vi "Engine Knocking Detection.vi"() -> ()   [LabVIEW 2023]
doc: "This example shows the application of arbitrary path decomposition in detecting engine knocking.\n\nAnalyzing the acoustic signals, or vibrations, of engines plays an important role in engine designing and testing. You can use the wavelet transform-based method to detect the knocking of an engine. In the example data, the knocking sound is merged in the noise. After processing the signal with wavelet-based arbitrary path decomposition and reconstruction, you can detect the knocking sound easily.\n\nThis example uses the WA Arbitrary Path Decomposition VI and the WA Arbitrary Path Reconstruction VI.\n\n<b>Instructions:</b>\n1) Run this VI.\n2) Observe how the engine knocking becomes obvious in the enhanced sound."
uses:
  <vilib>/addons/Wavelet Analysis/typedefs.llb/WA Data.ctl
  <vilib>/addons/Wavelet Analysis/discrete wavelet transform.llb/WA Arbitrary Path Decomposition (Waveform).vi
  <vilib>/addons/Wavelet Analysis/discrete wavelet transform.llb/WA Arbitrary Path Reconstruction (Waveform).vi
  <vilib>/addons/_Advanced Signal Processing/NI_AdvSigProcWA.lvlib
panel:
  out "aspt-left-top":bool
  in  "stop":bool
  in  "Path":string="11"
  in  "Wavelet":u16(ring) items=["db02"=0, "db03"=1, "db04"=2, "db05"=3, "db06"=4, "db07"=5, "db08"=6, "db09"=7, "db10"=8, "db11"=9, "db12"=10, "db13"=11, "db14"=12, "Haar"=13, "bior1_3"=14, "bior1_5"=15, "bior2_2"=16, "bior2_4"=17, "bior2_6"=18, "bior2_8"=19, "bior3_1"=20, "bior3_3"=21, "bior3_5"=22, "bior3_7"=23, "bior3_9"=24, "bior4_4 (FBI)"=25, "bior5_5"=38, "bior6_8"=39, "coif1"=26, "coif2"=27, "coif3"=28, "coif4"=29, "coif5"=30, "sym2"=31, "sym3"=32, "sym4"=33, "sym5"=34, "sym6"=35, "sym7"=36, "sym8"=37]
  out "Engine Knocking Sound":waveform(dbl)(graph)
  out "Enhanced Sound":waveform(dbl)(graph)
  # "Overview: Shows the application of arbitrary path decomposition in detecting engine knocking.\nRequirements: LabVIEW Full Development System, Advanced Signal Processing Toolkit\nInstructions: \n1. Run this VI.\n2. Observe how the engine knocking becomes obvious in the enhanced sound.\n3. Click Stop to stop the VI."
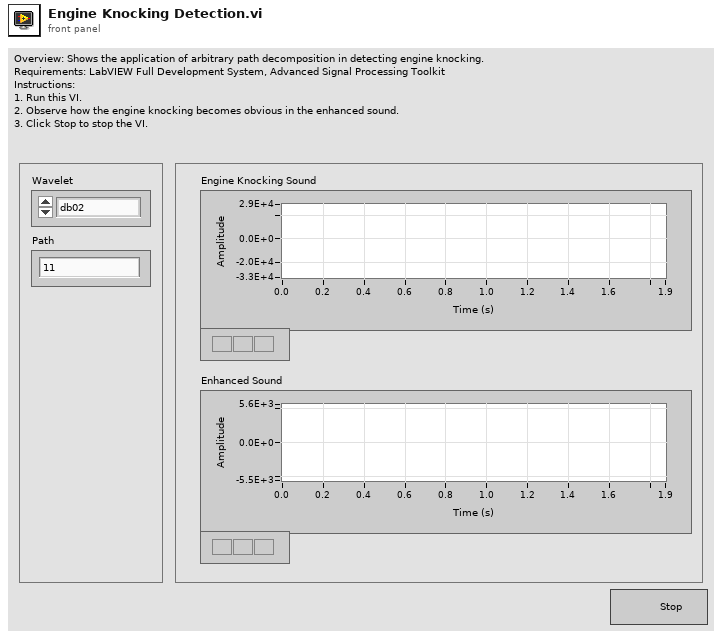
[diagram p1: front panel]
types:
  T1 = typedef "NI_AdvSigProcWA.lvlib/WA Data.ctl" = u16
  T2 = cluster{"coef":dbl[], "length":i32[], "residual path":string[]}
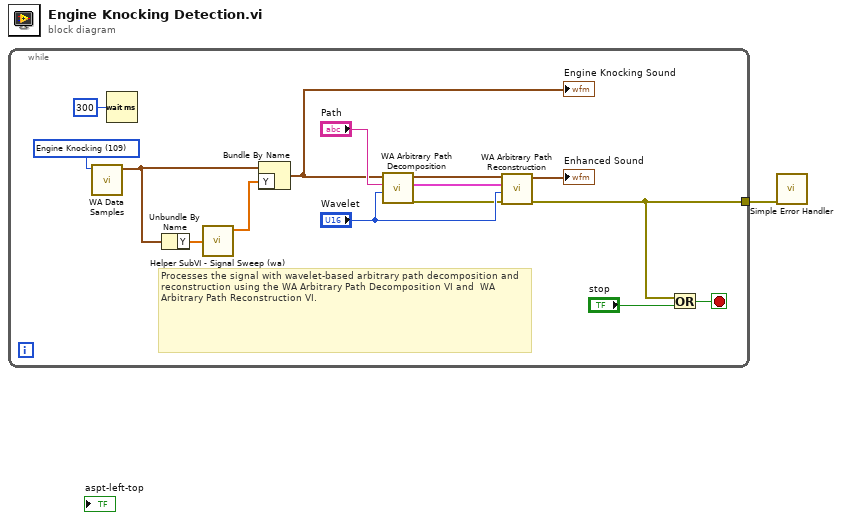
[diagram p0: block diagram]
diagram:
  n1 = while {
    tunnel: [w6] -> w1
    stop <- w9 stop-if-true
    w7 = T1 109 items=["1D Example Data"=100, "-"=101, "Doppler"=102, "HOP"=103, "TF Sine"=104, "Noisy Doppler"=105, "Sea Temperature"=106, "Sp500"=107, "Power Line"=108, "Engine Knocking"=109, "HeaviSine"=110, "Bumps"=111, "Blocks"=112, "Piece Regular"=113, "HypChirps"=114, "LinChirps"=115, "Chirps"=116, "Piece Polynomial"=117, "ECG"=131, "-"=118, "2D Example Data"=119, "-"=120, "Finger Print (Image)"=121, "Iris Flower (Image)"=122, "Mammogram (Image)"=123, "Lake (Image)"=127, "Two Can 1 (Image)"=132, "Two Can 2 (Image)"=133, "Camera Man (Image)"=134] ("data")
    # "Processes the signal with wavelet-based arbitrary path decomposition and reconstruction using the WA Arbitrary Path Decomposition VI and  WA Arbitrary Path Reconstruction VI."
    n2 = call <vilib>:"WA Data Samples.vi"("data"=w7) -> ("signal"=w3:waveform(dbl))  [unwired: 10 out]
    n3 = Wait (ms)(milliseconds to wait=u32 300 ("millisecond multiple")) -> ()  [unwired: 1 out]
    n4 = Unbundle By Name(w3) -> ("Y"=w5:dbl[])
    n5 = call "Helper SubVI - Signal Sweep (wa).vi"("Signal in"=w5) -> ("Signal out"=w4:dbl[])  [unwired: 10 in]
    n6 = Bundle By Name(cluster=w3, "Y"=w4) -> (w2:waveform(dbl))
    "Engine Knocking Sound" <- w2
    n7 = call-poly <vilib>:"WA Arbitrary Path Decomposition.vi"("wavelet"="Wavelet", "path"="Path", "signal"=w2) -> ("error out"=w11:errorcluster, "residual info"=w15:T2, "path coef"=w16:waveform(dbl))  [unwired: 1 in, 5 out]
    n8 = call-poly <vilib>:"WA Arbitrary Path Reconstruction.vi"("error in (no error)"=w11, "wavelet"="Wavelet", "residual info"=w15, "path coef"=w16) -> ("error out"=w6:errorcluster, "signal"=→"Enhanced Sound":waveform(dbl))  [unwired: 1 in, 5 out]
    n9 = Or(x=w6, y="stop") -> (x .or. y?=w9:bool)
  }
  n10 = call <vilib>:"Simple Error Handler.vi"("error in (no error)"=w1) -> ()  [unwired: 1 in, 8 out]
